vi "Pauli-X.vi"   [LabVIEW 2020]
doc: "Pauli-X Gate\n\nApplies a bit-flip (NOT). \nMaps |0> to |1> and |1> to |0>. \nRotates by pi radians around the X-axis. \n\nMatrix: [[ 0, 1], [ 1, 0]]"
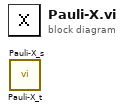
[diagram p0: block diagram]
diagram:
  n1 = call "Pauli-X_t.vi"() -> ()  [unwired: 15 in, 1 out]
  n2 = call "Pauli-X_s.vi"() -> ()  [unwired: 15 in, 1 out]
